vi "PathSupReindex.vi"(11 "PathSupremes":T1[](array[typedef])) -> (3 "PathSupOut":T1[](array[typedef]))   [LabVIEW 2014]
uses:
  TypeDefs/PathSupreme.ctl
  Sub/VelocityProfile.ctl
  Sub/PathCut.ctl
  Sub/Segment.ctl
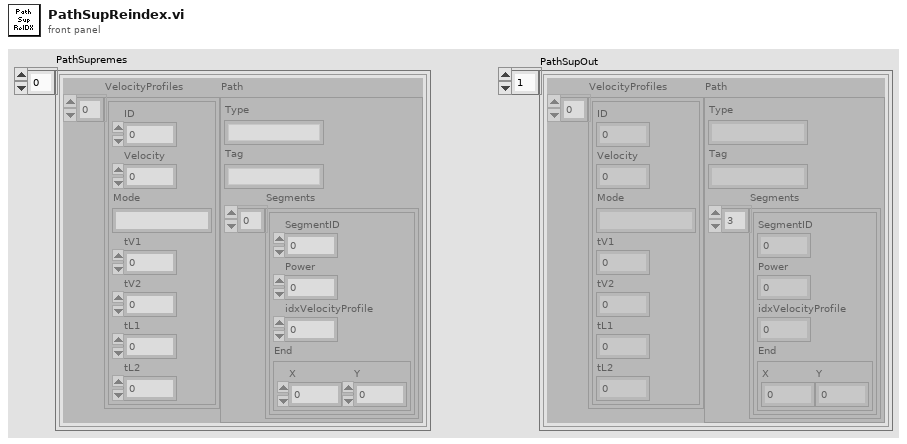
[diagram p1: front panel]
types:
  T1 = typedef "PathSupreme.ctl" = cluster{"VelocityProfiles":T2[], "Path":T3}
  T2 = typedef "VelocityProfile.ctl" = cluster{"ID":u32, "Velocity":dbl, "Mode":string, "tV1":u32, "tV2":u32, "tL1":u32, "tL2":u32}
  T3 = typedef "PathCut.ctl" = cluster{"Type":string, "Tag":string, "Segments":T4[]}
  T4 = typedef "Segment.ctl" = cluster{"SegmentID":u16, "Power":sgl, "idxVelocityProfile":u16, "End":cluster{"X":sgl, "Y":sgl}}
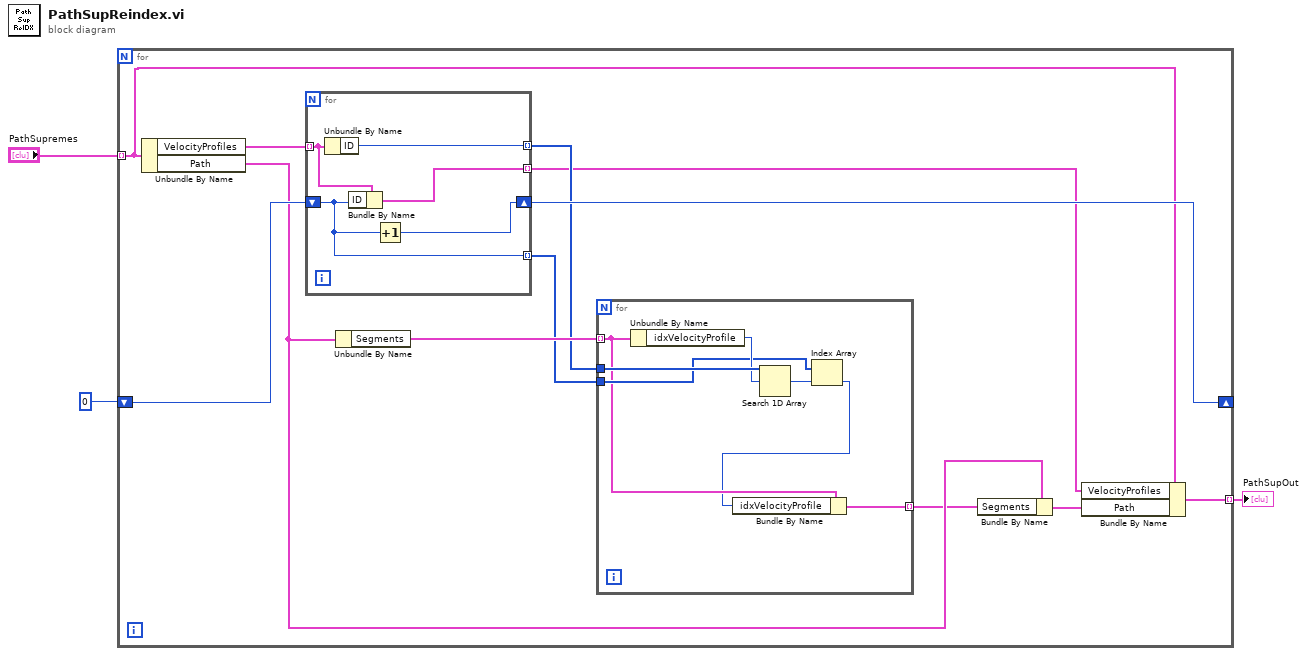
[diagram p0: block diagram]
diagram:
  n1 = for {
    shift-right: [w13] -> _
    shift-left: 0 -> [w14]
    tunnel: "PathSupremes" -> [w7] mode=indexing
    tunnel: [w4] -> w1 mode=indexing
    n2 = Unbundle By Name(w7) -> ("VelocityProfiles"=w15:T2[], "Path"=w9:T3)
    n3 = for {
      tunnel: w15 -> [w26] mode=indexing
      tunnel: [w27] -> w10 mode=indexing
      shift-right: [w25] -> w13
      shift-left: w14 -> [w23]
      tunnel: [w24] -> w5 mode=indexing
      tunnel: [w23] -> w11 mode=indexing
      n4 = Unbundle By Name(w26) -> ("ID"=w27:u32)
      n5 = Bundle By Name(cluster=w26, "ID"=w23) -> (w24:T2)
      n6 = Increment(x=w23) -> (x+1=w25:i32)
    }
    n7 = Unbundle By Name(w9) -> ("Segments"=w12:T4[])
    n8 = for {
      tunnel: w12 -> [w18] mode=indexing
      tunnel: w11 -> [w20]
      tunnel: w10 -> [w22]
      tunnel: [w16] -> w8 mode=indexing
      n9 = Unbundle By Name(w18) -> ("idxVelocityProfile"=w21:u16)
      n10 = Search 1D Array(1D array=w22, element=w21) -> (index of element=w19:i32)  [unwired: 1 in]
      n11 = Index Array(array=w20, index=w19) -> (element=w17:i32)
      n12 = Bundle By Name(cluster=w18, "idxVelocityProfile"=w17) -> (w16:T4)
    }
    n13 = Bundle By Name(cluster=w9, "Segments"=w8) -> (w6:T3)
    n14 = Bundle By Name(cluster=w7, "VelocityProfiles"=w5, "Path"=w6) -> (w4:T1)
  }
  "PathSupOut" <- w1
